vi "Set panel size and  place center.vi"(0 "Path":path, 1 "Close Reference (false)":bool, 2 "FP.WinOrigin in(H & V)":cluster{"Horizontal":i16, "Vertical":i16}, 5 "Panel Width":i32, 7 "Panel Height":i32, 9 "FP.Origin in(H & V)":cluster{"Horizontal":i16, "Vertical":i16}, 11 "error in (no error)":errorcluster, 12 "Set (false)":bool) -> (4 "Application or VI Refnum":refnum<vi>, 15 "error out":errorcluster)   [LabVIEW 2016]
doc: "This VI is used to set the panel size and plce it in the center of the window current"
uses:
  <vilib>/Utility/miscctls.llb/LVRectTypeDef.ctl
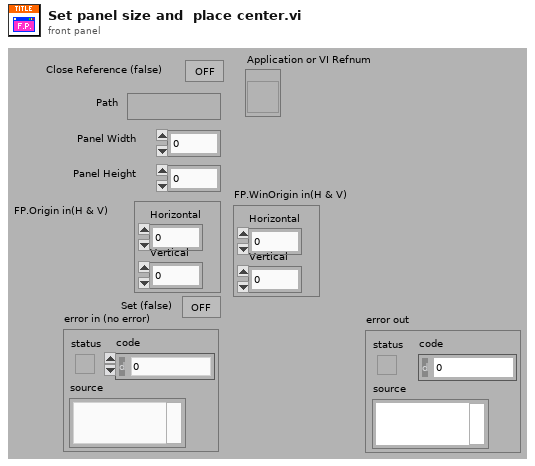
[diagram p1: front panel]
types:
  T1 = typedef "LVRectTypeDef.ctl" = cluster{"Left":i16, "Top":i16, "Right":i16, "Bottom":i16}
  T2 = typedef "LVAllMonitorsDisplayTypeDef.ctl" = cluster{"Bounds":cluster{"Left":i16, "Top":i16, "Right":i16, "Bottom":i16}, "Depth":i16}[]
  T3 = cluster{"Bounds":cluster{"Left":i16, "Top":i16, "Right":i16, "Bottom":i16}, "Depth":i16}
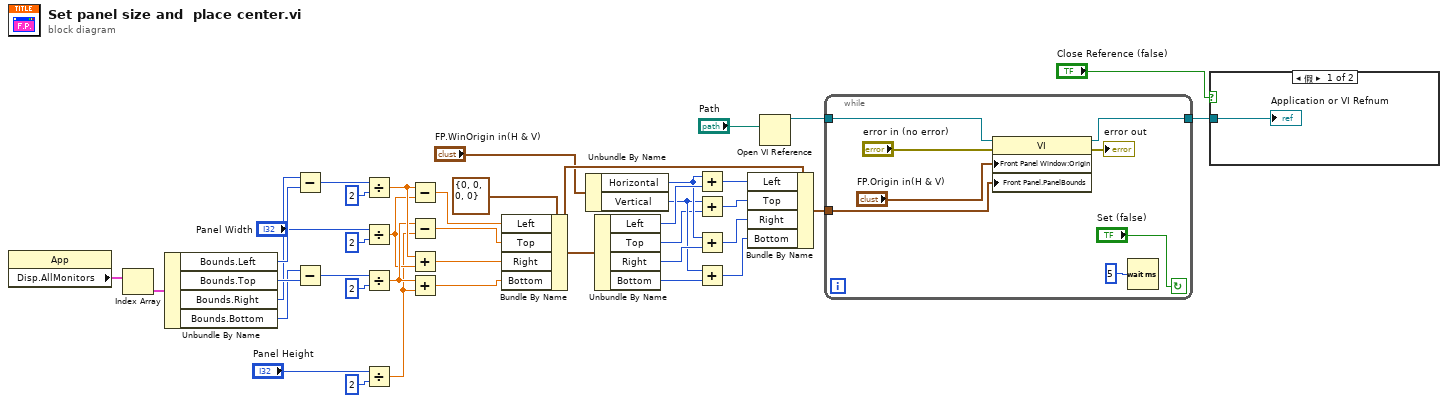
[diagram p0: block diagram]
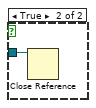
[diagram p2: hidden frame]
diagram:
  n1 = property class="App"() -> ("Disp.AllMonitors"=w15:T2)  [unwired: 2 in, 2 out]
  n2 = Index Array(array=w15) -> (element=w14:T3)  [unwired: 1 in]
  n3 = Unbundle By Name(w14) -> ("Bounds.Left"=w40:i16, "Bounds.Top"=w39:i16, "Bounds.Right"=w38:i16, "Bounds.Bottom"=w37:i16)
  n4 = Subtract(x=w38, y=w40) -> (x-y=w36:i16)
  n5 = Subtract(x=w37, y=w39) -> (x-y=w34:i16)
  n6 = Divide(x=w36, y=i16 2) -> (x/y=w28:dbl)
  n7 = Divide(x="Panel Width", y=2) -> (x/y=w26:dbl)
  n8 = Divide(x=w34, y=i16 2) -> (x/y=w27:dbl)
  n9 = Divide(x="Panel Height", y=2) -> (x/y=w25:dbl)
  n10 = Subtract(x=w28, y=w26) -> (x-y=w24:dbl)
  n11 = Subtract(x=w27, y=w25) -> (x-y=w22:dbl)
  n12 = Add(x=w28, y=w26) -> (x+y=w21:dbl)
  n13 = Add(x=w27, y=w25) -> (x+y=w23:dbl)
  n14 = Bundle By Name(cluster=T1 {"Left"=0, "Top"=0, "Right"=0, "Bottom"=0} ("显示:主工作区"), "Left"=w24, "Top"=w22, "Right"=w21, "Bottom"=w23) -> (w13:T1)
  n15 = Unbundle By Name("FP.WinOrigin in(H & V)") -> ("Horizontal"=w9:i16, "Vertical"=w5:i16)
  n16 = Unbundle By Name(w13) -> ("Left"=w11:i16, "Top"=w2:i16, "Right"=w8:i16, "Bottom"=w4:i16)
  n17 = Add(x=w9, y=w11) -> (x+y=w10:i16)
  n18 = Add(x=w5, y=w2) -> (x+y=w6:i16)
  n19 = Add(x=w9, y=w8) -> (x+y=w7:i16)
  n20 = Add(x=w5, y=w4) -> (x+y=w3:i16)
  n21 = Bundle By Name(cluster=w13, "Left"=w10, "Top"=w6, "Right"=w7, "Bottom"=w3) -> (w1:T1)
  n22 = Open VI Reference(vi path="Path") -> (vi reference=w20:refnum<vi>)  [unwired: 5 in, 1 out]
  n23 = while {
    tunnel: [w48] -> w17
    tunnel: w20 -> [w47]
    tunnel: w1 -> [w41]
    stop <- "Set (false)" continue-if-true
    n24 = property class="VI"(reference=w47, error in="error in (no error)", "Front Panel Window:Origin"="FP.Origin in(H & V)", "Front Panel.PanelBounds"=w41) -> (reference out=w48:refnum<vi>, error out=→"error out":errorcluster)
    n25 = Wait (ms)(milliseconds to wait=u32 5) -> ()  [unwired: 1 out]
  }
  n26 = case shown="假" "Close Reference (false)" {
    tunnel: w17 -> [w49 w50]
    frame False {
      "Application or VI Refnum" <- w49
    }
    frame True {
      n27 = Close Reference(reference=w50) -> ()  [unwired: 1 in, 1 out]
    }
  }
